vi "Backfil_pressure_Control.vi"() -> ()   [LabVIEW 2015]
uses:
  <vilib>/Utility/config.llb/Read Key (String).vi
  <vilib>/Instr/_visa.llb/VISA Configure Serial Port (Instr).vi
  <vilib>/Utility/config.llb/Read Key (Path).vi
  <vilib>/Utility/file.llb/Read From Spreadsheet File (DBL).vi
  <vilib>/Utility/config.llb/NI_LVConfig.lvlib
panel:
  in  "Boolean":bool
  in  "Enter the Set Point for the Flow":string
  in  "Please Close the Program After \nSetting the Flow":bool
  out "Acknowledgement":string
  out "Separator Flow":cluster{dbl[], dbl[]}(graph)
  in  "close":bool
  in  "open":bool
  out "error out 2":errorcluster
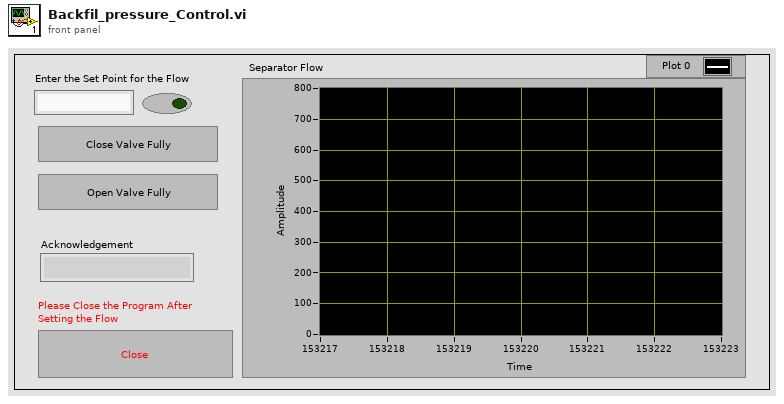
[diagram p1: front panel]
types:
  T1 = typedef "NI_LVConfig.lvlib/Config Data RefNum.ctl" = refnum<k1>
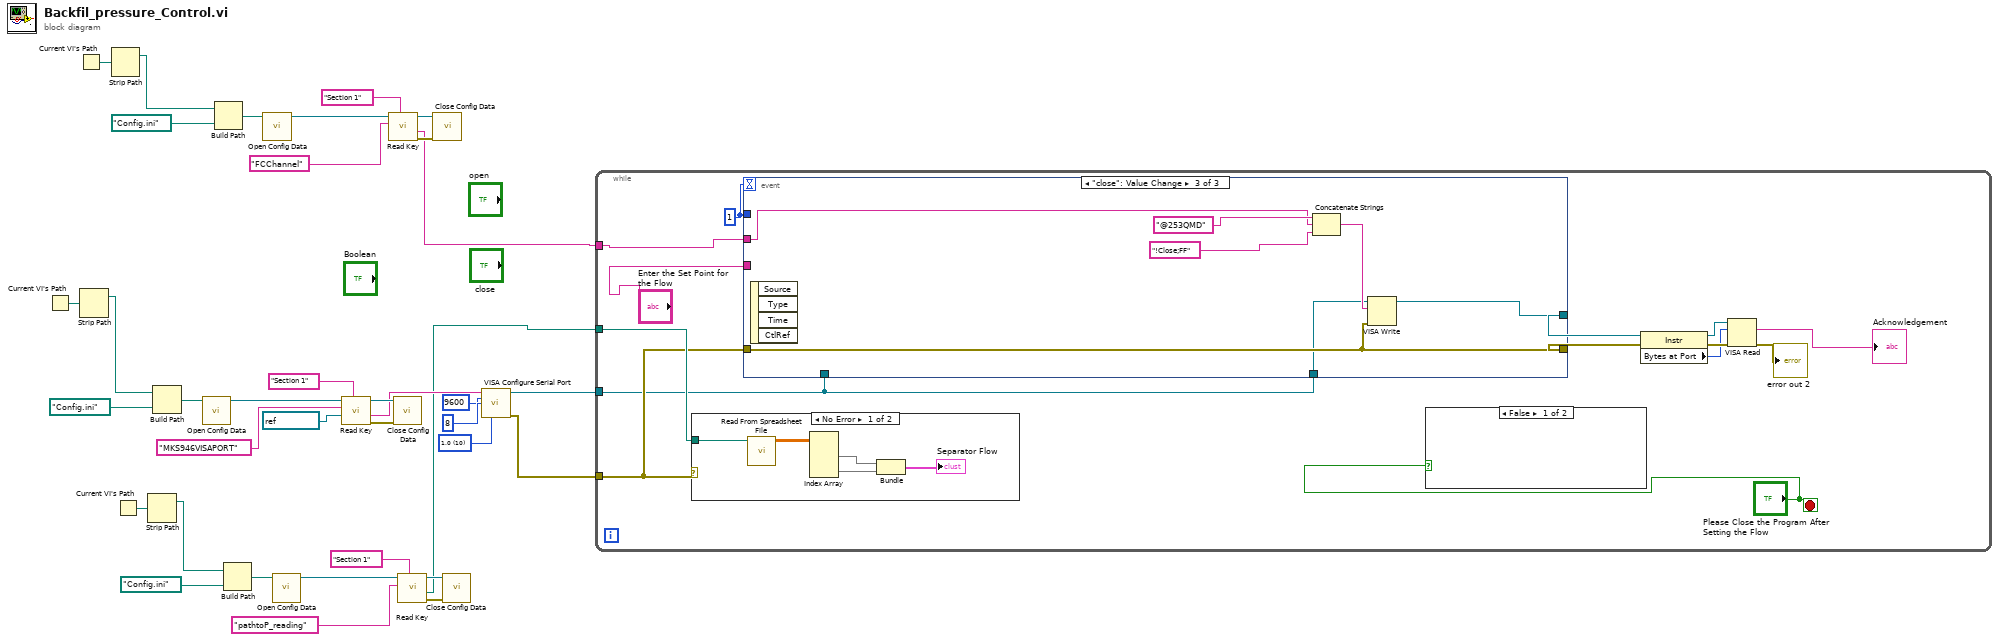
[diagram p0: block diagram]
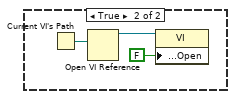
[diagram p2: hidden frame]
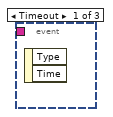
[diagram p3: hidden frame]
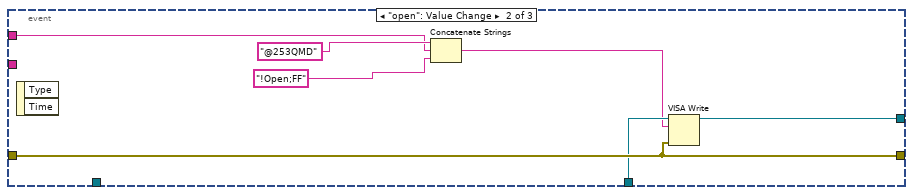
[diagram p4: hidden frame]
diagram:
  w34 = u16 10 items=["1.0"=10, "1.5"=15, "2.0"=20] ("stop bits (10: 1 bit)")
  n1 = Current VI's Path() -> (path=w4:path)
  n2 = Current VI's Path() -> (path=w6:path)
  n3 = Strip Path(path=w4) -> (stripped path=w3:path)  [unwired: 1 out]
  n4 = Strip Path(path=w6) -> (stripped path=w5:path)  [unwired: 1 out]
  n5 = Current VI's Path() -> (path=w2:path)
  n6 = Strip Path(path=w2) -> (stripped path=w1:path)  [unwired: 1 out]
  n7 = Build Path(base path=w3, name or relative path=path "Config.ini" ("default name")) -> (appended path=w28:path)
  n8 = call <vilib>:"Open Config Data.vi"("configuration file path"=w28) -> ("refnum"=w33:T1)  [unwired: 8 in, 2 out]
  n9 = Build Path(base path=w5, name or relative path=path "Config.ini" ("default name")) -> (appended path=w9:path)
  n10 = Build Path(base path=w1, name or relative path=path "Config.ini" ("default name")) -> (appended path=w19:path)
  n11 = call <vilib>:"Open Config Data.vi"("configuration file path"=w9) -> ("refnum"=w14:T1)  [unwired: 8 in, 2 out]
  n12 = call <vilib>:"Open Config Data.vi"("configuration file path"=w19) -> ("refnum"=w24:T1)  [unwired: 8 in, 2 out]
  n13 = call-poly <vilib>:"Read Key.vi"("section"="Section 1", "default value"=refnum<visa-resource-name> "COM5" ("VISA resource name"), "key"="MKS946VISAPORT", "refnum"=w33) -> ("error out"=w27:errorcluster, "value"=w25:string, "refnum out"=w31:T1)  [unwired: 4 in, 1 out]
  n14 = call-poly <vilib>:"Read Key.vi"("section"="Section 1", "key"="FCChannel", "refnum"=w14) -> ("error out"=w8:errorcluster, "value"=w7:string, "refnum out"=w12:T1)  [unwired: 5 in, 1 out]
  n15 = call <vilib>:"Close Config Data.vi"("error in (no error)"=w27, "refnum"=w31) -> ()  [unwired: 8 in, 2 out]
  n16 = call-poly <vilib>:"Read Key.vi"("section"="Section 1", "key"="pathtoP_reading", "refnum"=w24) -> ("error out"=w18:errorcluster, "value"=w17:path, "refnum out"=w22:T1)  [unwired: 5 in, 1 out]
  n17 = call <vilib>:"Close Config Data.vi"("error in (no error)"=w8, "refnum"=w12) -> ()  [unwired: 8 in, 2 out]
  n18 = call <vilib>:"Close Config Data.vi"("error in (no error)"=w18, "refnum"=w22) -> ()  [unwired: 8 in, 2 out]
  n19 = call-poly "VISA Configure Serial Port"("VISA resource name"=w25, "baud rate (9600)"=u32 9600, "data bits (8)"=u16 8, "stop bits (10: 1 bit)"=w34) -> ("VISA resource name out"=w15:refnum<visa-resource-name>, "error out"=w16:errorcluster)  [unwired: 10 in]
  n20 = while {
    tunnel: w17 -> [w50]
    tunnel: w16 -> [w45]
    tunnel: w15 -> [w37]
    tunnel: w7 -> [w41]
    stop <- "Please Close the Program After \nSetting the Flow" stop-if-true
    w46 = 1
    n21 = case shown="No Error" w45 {
      tunnel: w50 -> [w72 _]
      frame No Error {
        n22 = call-poly <vilib>:"Read From Spreadsheet File.vi"("file path (dialog if empty)"=w72) -> ("all rows"=w68:dbl[][])  [unwired: 6 in, 4 out]
        n23 = Index Array(array=w68) -> (element #1=w71:dbl[], element #2=w70:dbl[])  [unwired: 4 in]
        n24 = Bundle("all rows"=w71, "all rows"=w70) -> (→"Separator Flow":cluster{"all rows":dbl[], "all rows":dbl[]})  [unwired: 1 in]
      }
      frame Error {
      }
    }
    n25 = event shown="[2] \"close\": Value Change" {
      selector: _ -> [_ _ _]
      dyn-events: _ -> [_ _ _]
      timeout: w46 -> [_ _ _]
      tunnel: w46 -> [_ _ _]
      tunnel: w45 -> [_ w57 w64]
      tunnel: [_ w57 w64] -> w38
      tunnel: "Enter the Set Point for the Flow" -> [_ _ _]
      tunnel: w41 -> [_ w58 w65]
      tunnel: w37 -> [_ w56 w62]
      tunnel: [_ w54 w61] -> w39
      tunnel: w37 -> [_ _ _]
      event Timeout {
        n26 = event-data() -> ()  [unwired: 1 in, 2 out]
      }
      event "open": Value Change {
        n27 = event-data() -> ()  [unwired: 1 in, 2 out]
        n28 = Concatenate Strings("@253QMD", w58, "!Open;FF") -> (w55:string)
        n29 = VISA Write(VISA resource name=w56, write buffer=w55, error in (no error)=w57) -> (VISA resource name out=w54:refnum<visa-resource-name>)  [unwired: 2 out]
      }
      event "close": Value Change {
        n30 = event-data() -> ()  [unwired: 1 in, 4 out]
        n31 = Concatenate Strings("@253QMD", w65, "!Close;FF") -> (w63:string)
        n32 = VISA Write(VISA resource name=w62, write buffer=w63, error in (no error)=w64) -> (VISA resource name out=w61:refnum<visa-resource-name>)  [unwired: 2 out]
      }
    }
    n33 = case shown="False" "Please Close the Program After \nSetting the Flow" {
      frame False {
      }
      frame True {
        n34 = Current VI's Path() -> (path=w53:path)
        n35 = Open VI Reference(vi path=w53) -> (vi reference=w52:refnum<vi>)  [unwired: 5 in, 1 out]
        n36 = property class="VI"(reference=w52, "Front Panel Window:Open"=FALSE) -> ()  [unwired: 1 in, 2 out]
      }
    }
    n37 = property class="Instr"(reference=w39, error in=w38) -> (reference out=w47:refnum<visa-resource-name>, error out=w49:errorcluster, "Bytes at Port"=w48:u32)
    n38 = VISA Read(VISA resource name=w47, byte count=w48, error in (no error)=w49) -> (read buffer=→"Acknowledgement":string, error out=→"error out 2":errorcluster)  [unwired: 2 out]
  }
